vi "Set Error.vi"(10 "Error":errorcluster, 11 "Set Error in":refnum<class "Set Error.lvclass">) -> (3 "Set Error out":refnum<class "Set Error.lvclass">)   [LabVIEW 2021, in "Set Error.lvlib" / "Set Error.lvclass"]
uses:
  Set Error.lvclass
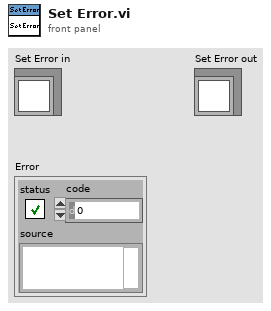
[diagram p1: front panel]
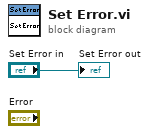
[diagram p0: block diagram]
diagram:
  "Set Error out" <- "Set Error in"
